vi "Module Timeout--constant.vi"() -> (3 "Module Timeout":i32)   [LabVIEW 2025, in "Torque Transducer.lvlib"]
doc: "A module-wide common value to use as the timeout for various synchronization actions.\n_____\nBased on DQMH Dev Tools: Project Template 7.1.2.1547."
uses:
  Torque Transducer.lvlib
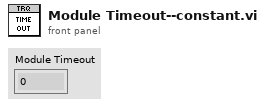
[diagram p1: front panel]
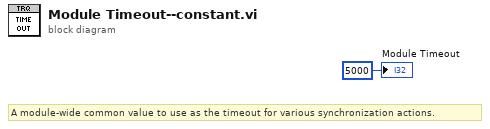
[diagram p0: block diagram]
diagram:
  # "A module-wide common value to use as the timeout for various synchronization actions."
  "Module Timeout" <- 5000 ("Module Timeout")
